vi "Read Calling VI Reference.vi"(11 "Philips Dialog in":refnum<class "Flex UI Dialog.lvclass">) -> (2 "Calling VI Reference":refnum<vi>, 3 "Philips Dialog out":refnum<class "Flex UI Dialog.lvclass">)   [LabVIEW 2014, in "Flex UI Dialog.lvclass"]
uses:
  Flex UI Dialog.lvclass
  Flex UI Dialog.lvclass/Flex UI Dialog.ctl
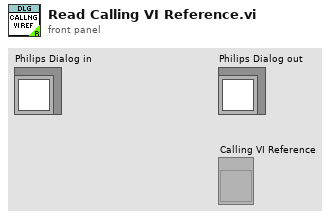
[diagram p1: front panel]
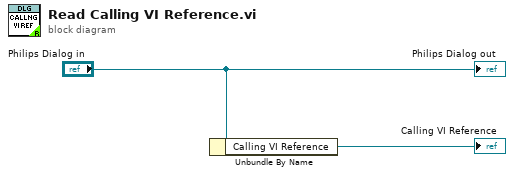
[diagram p0: block diagram]
diagram:
  n1 = Unbundle By Name("Philips Dialog in") -> ("Calling VI Reference"=→"Calling VI Reference":refnum<vi>)
  "Philips Dialog out" <- "Philips Dialog in"
